vi "Temperature-Main.vi"(8 "error int":errorcluster) -> (0 "error out":errorcluster)   [LabVIEW 2021]
doc: "Use this template to build a simple state machine design pattern. Each state executes code and determines which state to transition to."
uses:
  Controls/Temperature-State.ctl
  Controls/Temperature-Data.ctl
  Sensor-Class/Type-K-Thermocouple_class/Type-K-Thermocouple.lvclass
  Temperature-Module.lvlib
panel:
  out "Status":string
  out "Temperature":dbl[](array[numeric])
  in  "Run Display":bool
  in  "Exit":bool
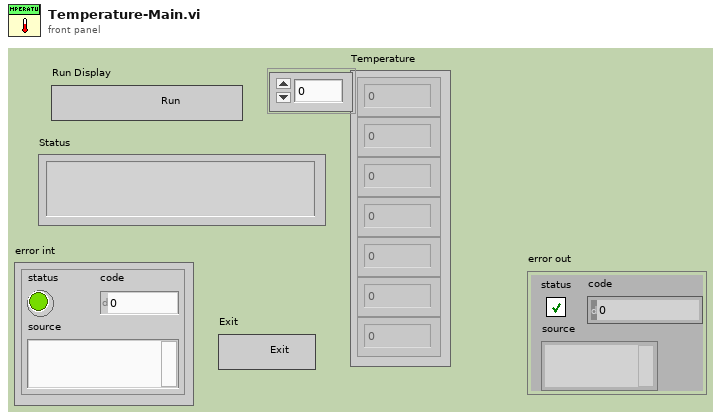
[diagram p1: front panel]
types:
  T1 = typedef "Temperature-Data.ctl" = cluster{"?":bool, "Status":string, "Temperature":dbl[], "Modbus-Instr":refnum<class "Type-K-Thermocouple.lvclass">}
  T2 = typedef "Temperature-State.ctl" = enum16{"Initialize", "Wait for Event", "Data: Run", "Data: Run-sym", "Data: Display", "Data: Close", "Error", "Exit"}
  T3 = typedef "Temperature-Module.lvlib/Request Events--cluster.ctl" = cluster{"Stop":refnum<user-event>, "Start Temp Display":refnum<user-event>}
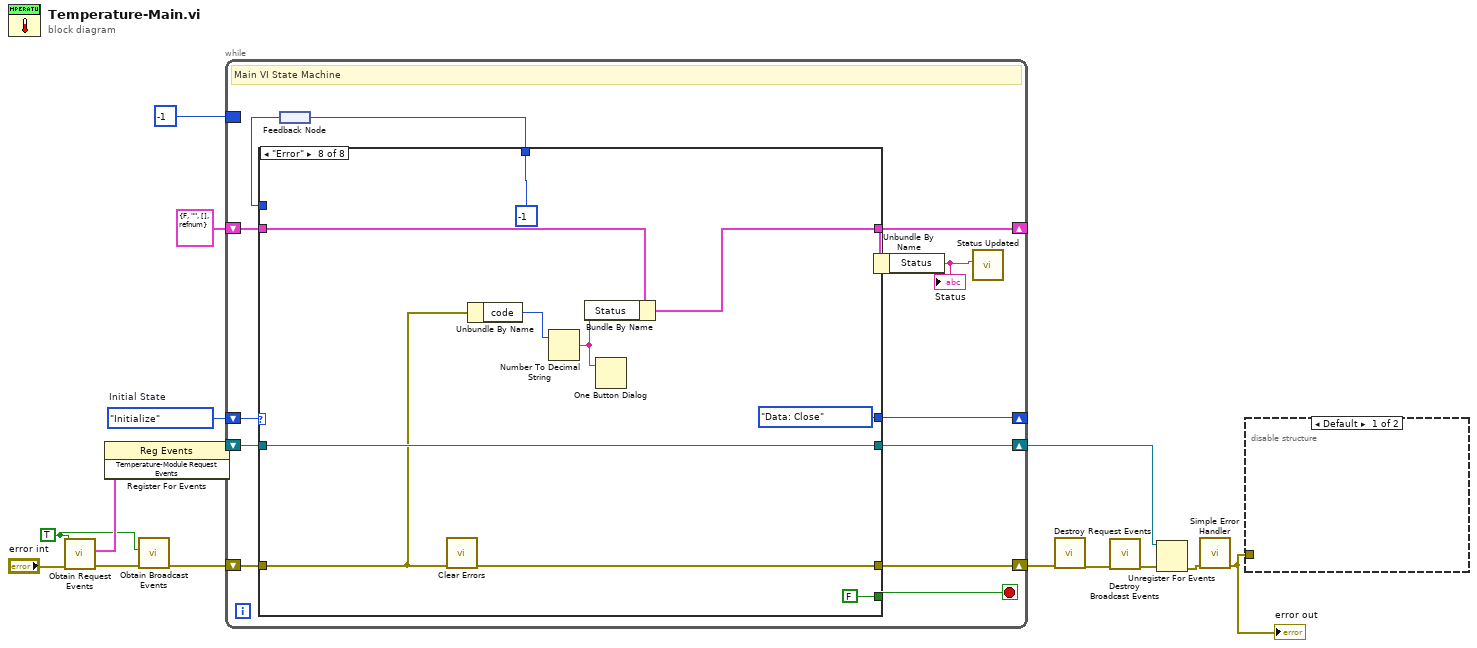
[diagram p0: block diagram]
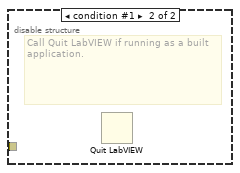
[diagram p2: hidden frame]
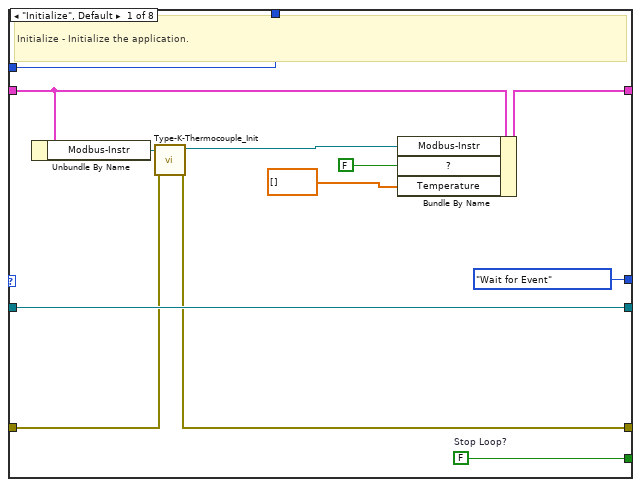
[diagram p3: hidden frame]
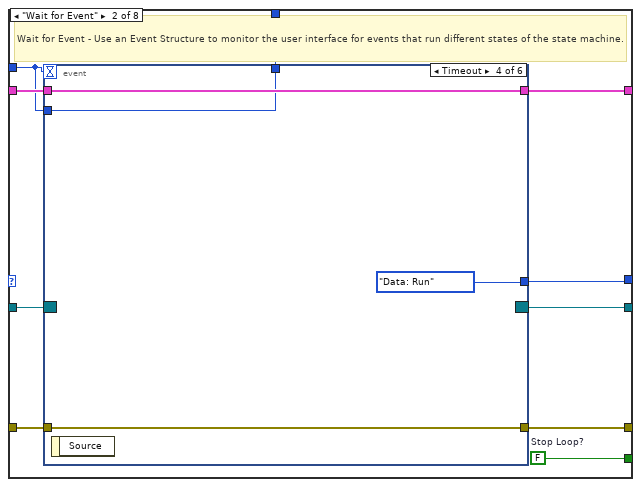
[diagram p4: hidden frame]
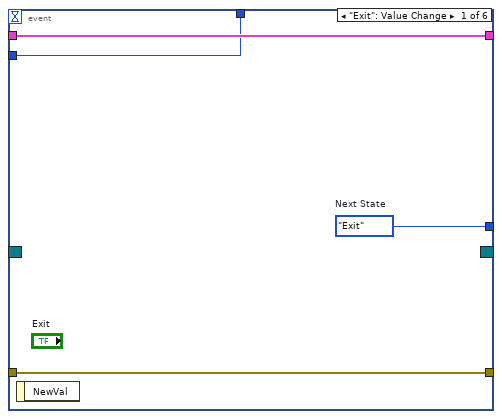
[diagram p5: hidden frame]
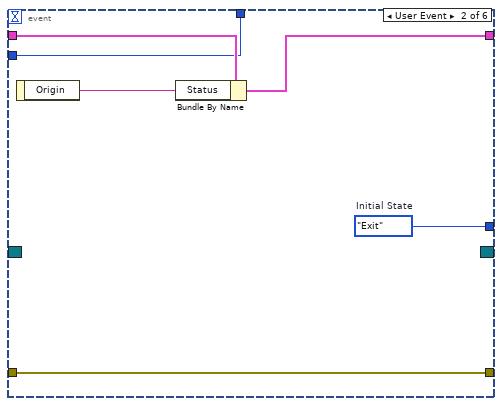
[diagram p6: hidden frame]
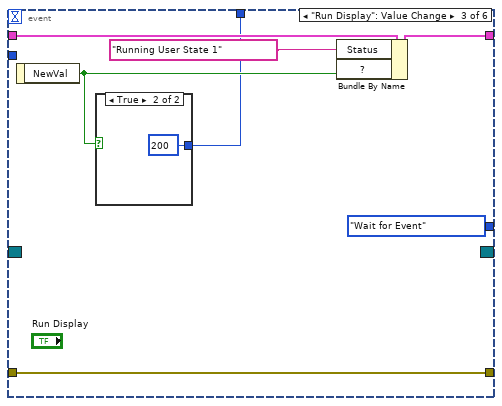
[diagram p7: hidden frame]
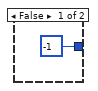
[diagram p8: hidden frame]
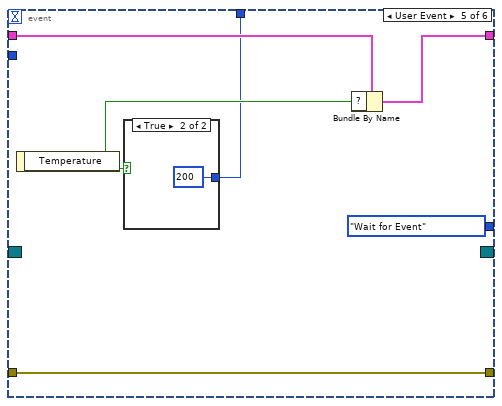
[diagram p9: hidden frame]
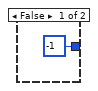
[diagram p10: hidden frame]
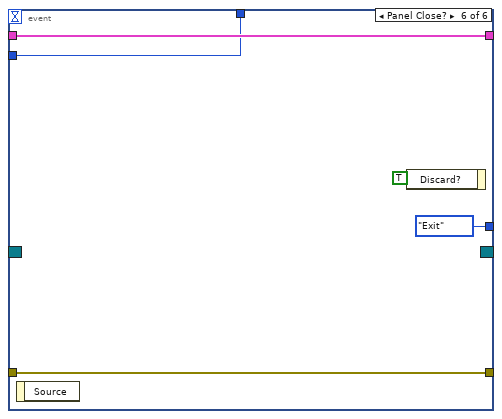
[diagram p11: hidden frame]
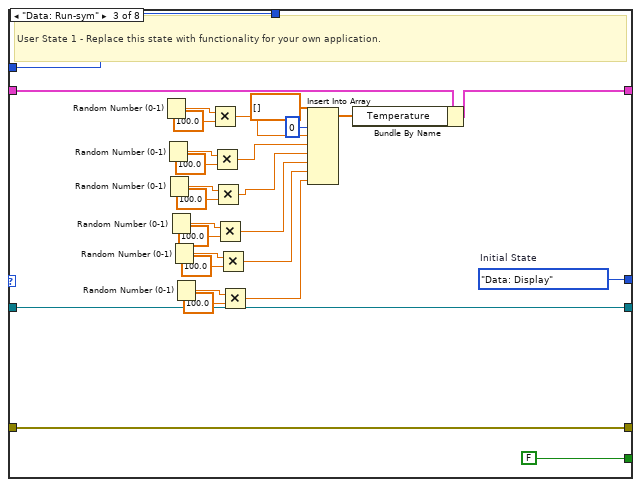
[diagram p12: hidden frame]
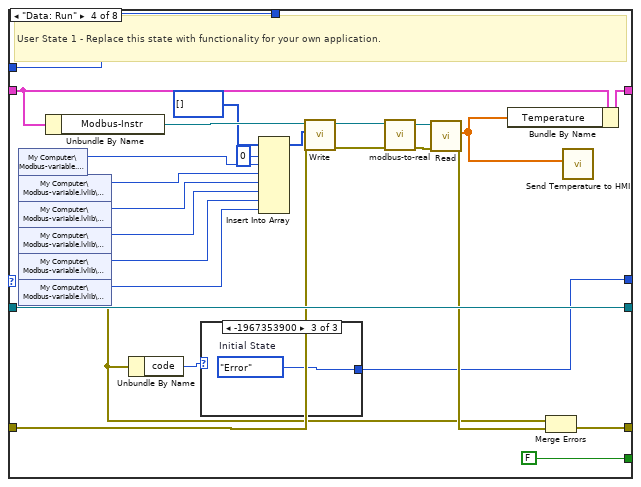
[diagram p13: hidden frame]
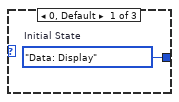
[diagram p14: hidden frame]
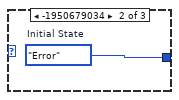
[diagram p15: hidden frame]
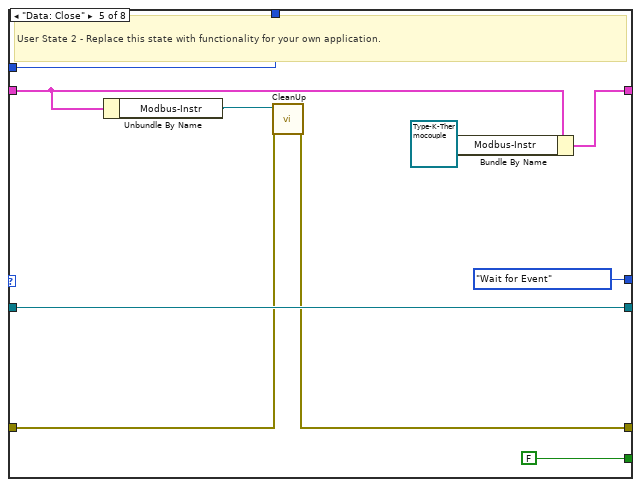
[diagram p16: hidden frame]
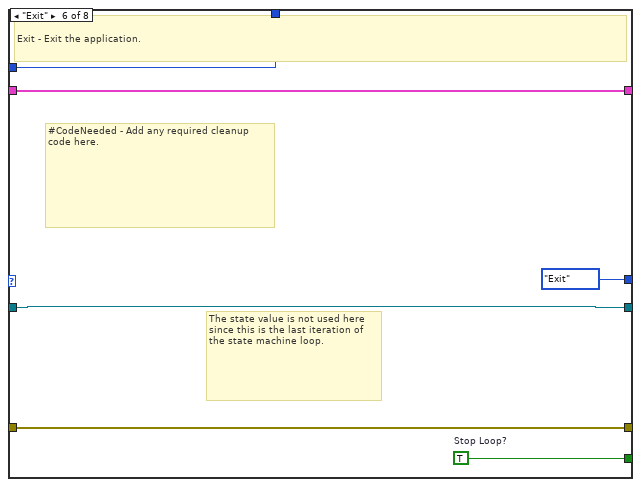
[diagram p17: hidden frame]
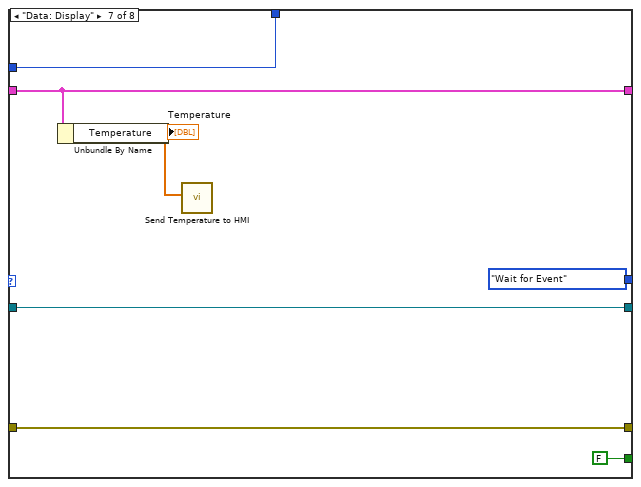
[diagram p18: hidden frame]
diagram:
  w8 = TRUE ("Create New?")
  w2 = Temperature-State."Initialize"  # Initial State
  n1 = call "Obtain Request Events.vi"("error in (no error)"="error int", "Create New?"=w8) -> ("error out"=w13:errorcluster, "Temperature-Module Request Events"=w9:T3)  [unwired: 8 in]
  n2 = register-events(w9) -> (reference out=w7:refnum<event-registration>)  [unwired: 2 in, 1 out]
  n3 = call "Obtain Broadcast Events.vi"("error in (no error)"=w13, "Create New?"=w8) -> ("error out"=w10:errorcluster)  [unwired: 8 in, 1 out]
  n4 = while {
    shift-right: [w21] -> _
    shift-left: T1 {"?"=FALSE, "Status"="", "Temperature"=[], "Modbus-Instr"=refnum} ("Data") -> [w27]
    shift-right: [w24] -> w5
    shift-left: w10 -> [w26]
    shift-right: [w22] -> w3
    shift-left: w7 -> [w23]
    shift-right: [w18] -> _
    shift-left: w2 -> [w19]
    border: -1 -> [_]
    stop <- w25 stop-if-true
    # "Main VI State Machine"
    n5 = feedback #1() -> (w17:i32)
    n6 = case shown="\"Error\"" w19 {
      tunnel: [w39 w49 FALSE ("Stop Loop?") FALSE ("Stop Loop?") FALSE ("Stop Loop?") w157 FALSE ("Stop Loop?") FALSE ("Stop Loop?")] -> w25
      tunnel: w27 -> [w33 w48 w107 w120 w146 w158 w163 w172]
      tunnel: [w38 w47 w106 w119 w145 w158 w163 w171] -> w21
      tunnel: w26 -> [w31 w46 w112 w125 w148 w156 w165 w170]
      tunnel: [w30 w45 w112 w128 w147 w156 w165 w166] -> w24
      tunnel: w23 -> [w36 w44 w111 w138 w151 w155 w164 w175]
      tunnel: [w36 w43 w111 w138 w151 w155 w164 w175] -> w22
      tunnel: [Temperature-State."Wait for Event" ("Initial State") w42 w110 w115 Temperature-State."Wait for Event" ("Initial State") Temperature-State."Exit" ("Initial State") Temperature-State."Wait for Event" ("Initial State") Temperature-State."Data: Close" ("Initial State")] -> w18
      tunnel: w17 -> [w28 w41 w86 w114 w143 w153 w159 _]
      tunnel: [w28 w40 w86 w114 w143 w153 w159 -1] -> w16
      frame "Initialize", Default {
        w39 = FALSE  # Stop Loop?
        # "Initialize - Initialize the application."
        n7 = Unbundle By Name(w33) -> ("Modbus-Instr"=w32:refnum<class "Type-K-Thermocouple.lvclass">)
        n8 = call "Type-K-Thermocouple_Init.vi"("error in (no error)"=w31, "object in"=w32) -> ("error out"=w30:errorcluster, "object out"=w29:refnum<class "Type-K-Thermocouple.lvclass">)  [unwired: 8 in]
        n9 = Bundle By Name(cluster=w33, "Modbus-Instr"=w29, "?"=FALSE ("Replace_Me_Boolean"), "Temperature"=dbl[] []) -> (w38:T1)
      }
      frame "Wait for Event" {
        w49 = FALSE  # Stop Loop?
        # "Wait for Event - Use an Event Structure to monitor the user interface for events that run different states of the state machine."
        n10 = event shown="[3] Timeout" {
          selector: w44 -> [_ _ _ _ _ _]
          dyn-events: [_ _ _ _ _ _] -> w43
          timeout: w41 -> [_ _ _ _ _ _]
          tunnel: [w53 w55 Temperature-State."Wait for Event" ("Initial State") Temperature-State."Data: Run" ("Initial State") Temperature-State."Wait for Event" ("Initial State") Temperature-State."Exit" ("Initial State")] -> w42
          tunnel: w48 -> [w52 w58 w66 w71 w77 w85]
          tunnel: [w52 w56 w65 w71 w76 w85] -> w47
          tunnel: w46 -> [w51 w59 w63 w72 w78 w84]
          tunnel: [w51 w59 w63 w72 w78 w84] -> w45
          tunnel: w41 -> [w50 w54 _ w69 _ w81]
          tunnel: [w50 w54 w60 w69 w73 w81] -> w40
          event "Exit": Value Change {
            w53 = Temperature-State."Exit"  # Next State
            n11 = event-data() -> ()  [unwired: 1 in, 1 out]
          }
          event User Event {
            w55 = Temperature-State."Exit"  # Initial State
            n12 = event-data() -> ("Origin"=w57:string)  [unwired: 1 in]
            n13 = Bundle By Name(cluster=w58, "Status"=w57) -> (w56:T1)
          }
          event "Run Display": Value Change {
            n14 = event-data() -> ("NewVal"=w61:bool)  [unwired: 1 in]
            n15 = case shown="True" w61 {
              tunnel: [-1 200] -> w60
              frame False {
              }
              frame True {
              }
            }
            n16 = Bundle By Name(cluster=w66, "Status"="Running User State 1" ("Running User State 1"), "?"=w61) -> (w65:T1)
          }
          event Timeout {
            n17 = event-data() -> ()  [unwired: 1 in, 1 out]
          }
          event User Event {
            n18 = event-data() -> ("Temperature"=w74:bool)  [unwired: 1 in]
            n19 = case shown="True" w74 {
              tunnel: [-1 200] -> w73
              frame False {
              }
              frame True {
              }
            }
            n20 = Bundle By Name(cluster=w77, "?"=w74) -> (w76:T1)
          }
          event Panel Close? {
            n21 = event-data() -> ()  [unwired: 1 in, 1 out]
            n22 = event-data("Discard?"=TRUE) -> ()  [unwired: 1 in, 1 out]
          }
        }
      }
      frame "Data: Run-sym" {
        w110 = Temperature-State."Data: Display"  # Initial State
        # "User State 1 - Replace this state with functionality for your own application."
        n23 = Random Number (0-1)() -> (number: 0 to 1=w109:dbl)
        n24 = Random Number (0-1)() -> (number: 0 to 1=w104:dbl)
        n25 = Random Number (0-1)() -> (number: 0 to 1=w103:dbl)
        n26 = Random Number (0-1)() -> (number: 0 to 1=w100:dbl)
        n27 = Random Number (0-1)() -> (number: 0 to 1=w96:dbl)
        n28 = Random Number (0-1)() -> (number: 0 to 1=w99:dbl)
        n29 = Multiply(x=w109, y=100.0) -> (x*y=w94:dbl)
        n30 = Multiply(x=w104, y=100.0) -> (x*y=w93:dbl)
        n31 = Multiply(x=w103, y=100.0) -> (x*y=w92:dbl)
        n32 = Multiply(x=w100, y=100.0) -> (x*y=w91:dbl)
        n33 = Multiply(x=w96, y=100.0) -> (x*y=w90:dbl)
        n34 = Multiply(x=w99, y=100.0) -> (x*y=w89:dbl)
        n35 = Insert Into Array(array=dbl[] [], index=0, new element #1=w94, new element #2=w93, new element #3=w92, new element #4=w91, new element #5=w90, new element #6=w89) -> (w87:dbl[])
        n36 = Bundle By Name(cluster=w107, "Temperature"=w87) -> (w106:T1)
      }
      frame "Data: Run" {
        # "User State 1 - Replace this state with functionality for your own application."
        n37 = shared-variable "My Computer\\Modbus-variable.lvlib\\T 1"() -> (w136:u16)  [unwired: 1 in, 1 out]
        n38 = shared-variable "My Computer\\Modbus-variable.lvlib\\400002"() -> (w133:u16)  [unwired: 1 in, 1 out]
        n39 = shared-variable "My Computer\\Modbus-variable.lvlib\\400003"() -> (w132:u16)  [unwired: 1 in, 1 out]
        n40 = shared-variable "My Computer\\Modbus-variable.lvlib\\400004"() -> (w131:u16)  [unwired: 1 in, 1 out]
        n41 = shared-variable "My Computer\\Modbus-variable.lvlib\\400005"() -> (w130:u16)  [unwired: 1 in, 1 out]
        n42 = shared-variable "My Computer\\Modbus-variable.lvlib\\400006"() -> (w129:u16, error out=w117:errorcluster)  [unwired: 1 in]
        n43 = Unbundle By Name(w120) -> ("Modbus-Instr"=w137:refnum<class "Type-K-Thermocouple.lvclass">)
        n44 = Unbundle By Name(w117) -> ("code"=w116:i32)
        n45 = case shown="-1967353900" w116 {
          tunnel: [w140 w141 w142] -> w115
          frame 0, Default {
            w140 = Temperature-State."Data: Display"  # Initial State
          }
          frame -1950679034 {
            w141 = Temperature-State."Error"  # Initial State
          }
          frame -1967353900 {
            w142 = Temperature-State."Error"  # Initial State
          }
        }
        n46 = Insert Into Array(array=u16[] [], index=0, new element #1=w136, new element #2=w133, new element #3=w132, new element #4=w131, new element #5=w130, new element #6=w129) -> (w127:u16[])
        n47 = call-dynamic "Write.vi"("error in (no error)"=w125, "Modbus-Reg"=w127, "object in"=w137) -> ("error out"=w126:errorcluster, "object out"=w124:refnum<class "Type-K-Thermocouple.lvclass">)  [unwired: 7 in]
        n48 = call-dynamic "modbus-to-real.vi"("error in (no error)"=w126, "object in"=w124) -> ("error out"=w122:errorcluster, "object out"=w123:refnum<class "Type-K-Thermocouple.lvclass">)  [unwired: 8 in]
        n49 = call-dynamic "Read.vi"("error in (no error)"=w122, "object in"=w123) -> ("error out"=w121:errorcluster, "Data"=w118:dbl[])  [unwired: 7 in, 1 out]
        n50 = Bundle By Name(cluster=w120, "Temperature"=w118) -> (w119:T1)
        n51 = Merge Errors(w117, w121) -> (w128:errorcluster)
        n52 = call "Send Temperature to HMI.vi"("Temperature"=w118) -> ()  [unwired: 10 in, 1 out]
      }
      frame "Data: Close" {
        # "User State 2 - Replace this state with functionality for your own application."
        n53 = Unbundle By Name(w146) -> ("Modbus-Instr"=w149:refnum<class "Type-K-Thermocouple.lvclass">)
        n54 = call-dynamic "CleanUp.vi"("error in (no error)"=w148, "object in"=w149) -> ("error out"=w147:errorcluster)  [unwired: 8 in, 1 out]
        n55 = Bundle By Name(cluster=w146, "Modbus-Instr"=refnum<class "Type-K-Thermocouple.lvclass"> refnum) -> (w145:T1)
      }
      frame "Exit" {
        w157 = TRUE  # Stop Loop?
        # "#CodeNeeded - Add any required cleanup code here."
        # "The state value is not used here since this is the last iteration of the state machine loop."
        # "Exit - Exit the application."
      }
      frame "Data: Display" {
        n56 = Unbundle By Name(w163) -> ("Temperature"=w160:dbl[])
        "Temperature" <- w160
        n57 = call "Send Temperature to HMI.vi"("Temperature"=w160) -> ()  [unwired: 10 in, 1 out]
      }
      frame "Error" {
        n58 = call <vilib>:"Clear Errors.vi"("error in (no error)"=w170) -> ("error out"=w166:errorcluster)  [unwired: 5 in, 1 out]
        n59 = Unbundle By Name(w170) -> ("code"=w168:i32)
        n60 = Number To Decimal String(number=w168) -> (decimal integer string=w167:string)  [unwired: 1 in]
        n61 = Bundle By Name(cluster=w172, "Status"=w167) -> (w171:T1)
        n62 = One Button Dialog(message=w167) -> ()  [unwired: 1 in, 1 out]
      }
    }
    n63 = feedback-in #1(w16) -> ()
    n64 = Unbundle By Name(w21) -> ("Status"=w20:string)
    "Status" <- w20
    n65 = call "Status Updated.vi"("Status"=w20) -> ()  [unwired: 10 in, 1 out]
  }
  n66 = call "Destroy Request Events.vi"("error in (no error)"=w5) -> ("error out"=w12:errorcluster)  [unwired: 10 in]
  n67 = call "Destroy Broadcast Events.vi"("error in (no error)"=w12) -> ("error out"=w6:errorcluster)  [unwired: 10 in]
  n68 = Unregister For Events(event registration refnum=w3, error in=w6) -> (error out=w4:errorcluster)
  n69 = call <vilib>:"Simple Error Handler.vi"("error in (no error)"=w4) -> ("error out"=w14:errorcluster)  [unwired: 4 in, 4 out]
  "error out" <- w14
  n70 = disable-structure shown="Default" {
    disable-tunnel: w14 -> [_ _]
    frame condition #0 (active) {
    }
    frame condition #1 {
      # "Call Quit LabVIEW if running as a built application."
      n71 = Quit LabVIEW() -> ()  [unwired: 1 in]
    }
  }
